vi "PH_Class.panel.vi"(0 "object ref":refnum<vi>, 5 "error in (no error)":errorcluster) -> (19 "error out":errorcluster)   [LabVIEW 2014, in "PH_Class.lvlib"]
doc: "By this VI a hardware switch can be monitored and switched. \n\nThe indicators \"FALSE\", \"TRUE\" and \"SWITCH STATE\" show the value of the Beckhoff-Tag: blue indicates bad tag status reference problems, darkgreen false and lightgreen true. If everything is working fine, \"FALSE\" and \"SWITCH STATE\" should show the same value, while \"TRUE\" has the opposite value. The caption of the sensors for \"FALSE\" and \"TRUE\" are taken out of the database. In case of only one or no sensor these GUI elements are not shown at all.\n\nThe oval button switches. It should be in the same state as the \"SWITCH STATE\" indicator. \n\n\"Delete Instance\" disconnects and removes the instance from the PCS.\n\n\nLicense Agreement for this software:\n\nCopyright (C)\nGesellschaft für Schwerionenforschung, GSI\nPlanckstr. 1\n64291 Darmstadt\nGermany\n\nContact: D.Beck@gsi.de \n\nThis program is free software; you can redistribute it and/or modify it under the terms of the GNU General Public License as published by the Free Software Foundation; either version 2 of the license, or (at your option) any later version.\n\nThis program is distributed in the hope that it will be useful, but WITHOUT ANYW ARRANTY; without even the implied warranty of MERCHANTABILITY or FITNESS FOR A PARTICULAR PURPOSE. See the GNU General License for more details (http://www.gnu.org).\n\nGesellschaft für Schwerionenforschung, GSI\nPlanckstr. 1, 64291 Darmstadt, Germany\nFor all questions and ideas contact: M.Richter@gsi.de, H.Brand@gsi.de or D.Beck@gsi.de.\nLast update: 18-DEC-2002"
uses:
  PH_Class.lvlib
  PH_Common/PH_Common.lvlib
panel:
  in  "Delete":bool
  out "loop counter":i32
  # "PCS"
  # "3.40"
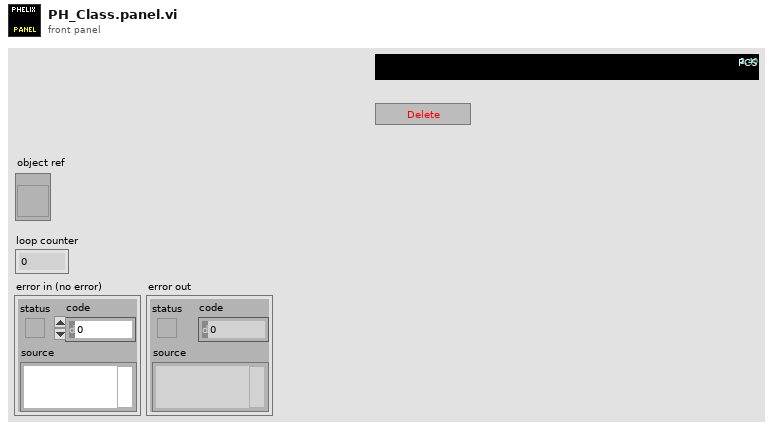
[diagram p1: front panel]
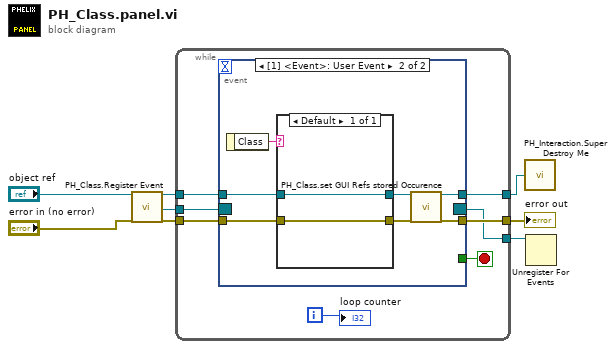
[diagram p0: block diagram]
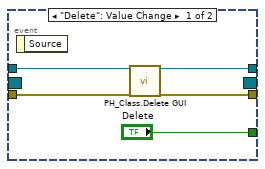
[diagram p2: hidden frame]
diagram:
  n1 = call "PH_Class.Register Event.vi"("i ref in"="object ref", "error in (no error)"="error in (no error)") -> ("i ref out"=w3:refnum<vi>, "Event Registration Refnum"=w2:refnum<event-registration>, "error out"=w4:errorcluster)  [unwired: 15 in]
  n2 = while {
    tunnel: w3 -> [w12]
    tunnel: [w11] -> w8
    tunnel: w4 -> [w14]
    tunnel: [w13] -> w7
    tunnel: w2 -> [w10]
    tunnel: [w9] -> w1
    i -> [w15]
    stop <- w16 stop-if-true
    n3 = event shown="[1] <Event>: User Event" {
      selector: w10 -> [_ _]
      dyn-events: [_ _] -> w9
      timeout: _ -> [_ _]
      tunnel: ["Delete" _] -> w16
      tunnel: w12 -> [w19 w28]
      tunnel: w14 -> [w20 w27]
      tunnel: [w17 w24] -> w13
      tunnel: [w18 w22] -> w11
      event "Delete": Value Change {
        n4 = event-data() -> ()  [unwired: 1 in, 1 out]
        n5 = call "PH_Class.Delete GUI.vi"("VI in"=w19, "error in (no error)"=w20) -> ("VI out"=w18:refnum<vi>, "error out"=w17:errorcluster)  [unwired: 16 in]
      }
      event User Event {
        n6 = event-data() -> ("Class"=w25:string)  [unwired: 1 in]
        n7 = case shown="Default" w25 {
          tunnel: w28 -> [w30]
          tunnel: [w30] -> w23
          tunnel: w27 -> [w29]
          tunnel: [w29] -> w26
          frame Default {
          }
        }
        n8 = call "PH_Class.set GUI Refs stored Occurence.vi"("i ref in"=w23, "error in (no error)"=w26) -> ("i ref out"=w22:refnum<vi>, "error out"=w24:errorcluster)  [unwired: 16 in]
      }
    }
    "loop counter" <- w15
  }
  "error out" <- w7
  n9 = call "PH_Interaction.Super Destroy Me.vi"("i ref out"=w8) -> ()
  n10 = Unregister For Events(event registration refnum=w1) -> ()  [unwired: 1 in, 1 out]
